vi "Read Generated files.vi"(8 "error in (no error)":errorcluster, 11 "Build Named Build Specification Data in":refnum<class "Build Named Build Specification Data.lvclass">) -> (0 "error out":errorcluster, 2 "Generated files":path[](array[path]), 3 "Build Named Build Specification Data out":refnum<class "Build Named Build Specification Data.lvclass">)   [LabVIEW 2020, in "ProjectBuilder.lvlib" / "Build Named Build Specification Data.lvclass"]
uses:
  Build Named Build Specification Data.lvclass
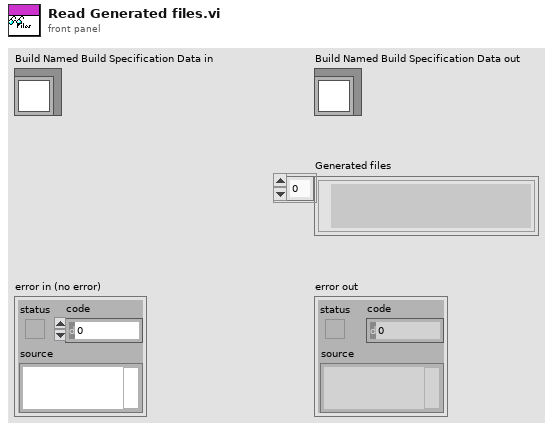
[diagram p1: front panel]
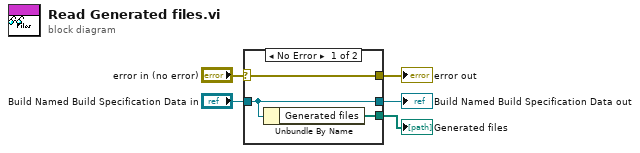
[diagram p0: block diagram]
diagram:
  n1 = case shown="No Error" "error in (no error)" {
    selector: "error in (no error)" -> [w8 w9]
    tunnel: [w8 w9] -> w4
    tunnel: [w7 w10] -> w2
    tunnel: "Build Named Build Specification Data in" -> [w7 w10]
    tunnel: [w6 _] -> w1
    frame No Error {
      n2 = Unbundle By Name(w7) -> ("Generated files"=w6:path[])
    }
    frame Error {
    }
  }
  "error out" <- w4
  "Build Named Build Specification Data out" <- w2
  "Generated files" <- w1
